vi "Self Configure.vi"(8 "error in":errorcluster, 11 "PowerSupply in":refnum<class "PowerSupply.lvclass">) -> (0 "error out":errorcluster, 3 "PowerSupply out":refnum<class "PowerSupply.lvclass">)   [LabVIEW 2019, in "PowerSupply.lvlib" / "PowerSupply.lvclass"]
uses:
  Library/PowerSupply.lvclass
  Custom Controls/Configuration Keys.ctl
  Library/PowerSupply.lvclass/PowerSupply.ctl
  builds/Instruments/Instruments.lvlibp/Library/Instruments.lvclass
  builds/Tools/Config.lvlibp/Config.lvclass
  C:/Users/Public/Documents/Development/builds/Instruments/Instruments.lvlibp/Library/Instruments.lvclass
  C:/Users/Public/Documents/Development/builds/Tools/Config.lvlibp/Config.lvclass
  C:/Users/Public/Documents/Development/builds/Engine/Engine.lvlibp/Project/Engine.lvclass
  C:/Users/Public/Documents/Development/builds/Engine/State Actor.lvlibp/Library/State Actor.lvclass
  C:/Users/Public/Documents/Development/builds/Engine/Panel Manager.lvlibp/Panel Actor/Panel Actor.lvclass
  C:/Users/Public/Documents/Development/builds/Engine/Monitored Actor.lvlibp/Monitored Actor/Monitored Actor/Monitored Actor.lvclass
  C:/Users/Public/Documents/Development/builds/Engine/Actor Framework.lvlibp/1abvi3w/vi.lib/ActorFramework/Actor/Actor.lvclass
panel:
  in  "Configuration Keys":T1
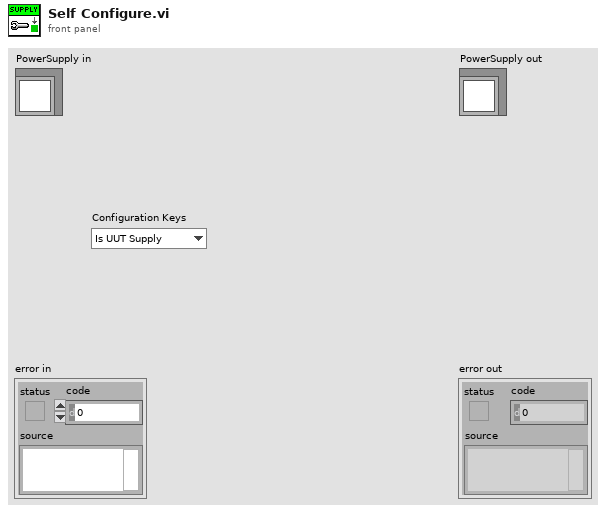
[diagram p1: front panel]
types:
  T1 = typedef "PowerSupply.lvlib/PowerSupply.lvclass/Configuration Keys.ctl" = enum16{"Is UUT Supply", "Number of Channels", "Channel Names", "Max Voltage", "Max Current", "Max OVP", "Max OCP", "Max Volt Ramp", "Max Curr Ramp"}
  T2 = typedef "PowerSupply.lvlib/PowerSupply.lvclass/Limits.ctl" = cluster{"Max_Current":dbl, "Max_Voltage":dbl, "Max_Current_Ramp":dbl, "Max_Voltage_Ramp":dbl, "Max_OCP":dbl, "Max_OVP":dbl}
  T3 = typedef "PowerSupply.lvlib/PowerSupply.lvclass/Settings.ctl" = cluster{"Voltage":dbl, "Current":dbl, "Output":bool, "OverVolt_Protect":dbl, "OverCurrent_Protect":dbl, "OVP":bool, "OCP":bool, "Interlock":bool, "Volt_Ramp":dbl, "Current_Ramp":dbl, "Sense Point":T4, "OCP Mode":T5, "Sharing":bool}
  T4 = typedef "PowerSupply.lvlib/PowerSupply.lvclass/Sense Point.ctl" = enum16{"Local", "Remote"}
  T5 = typedef "PowerSupply.lvlib/PowerSupply.lvclass/OCP Mode.ctl" = enum16{"Shutdown", "Foldback"}
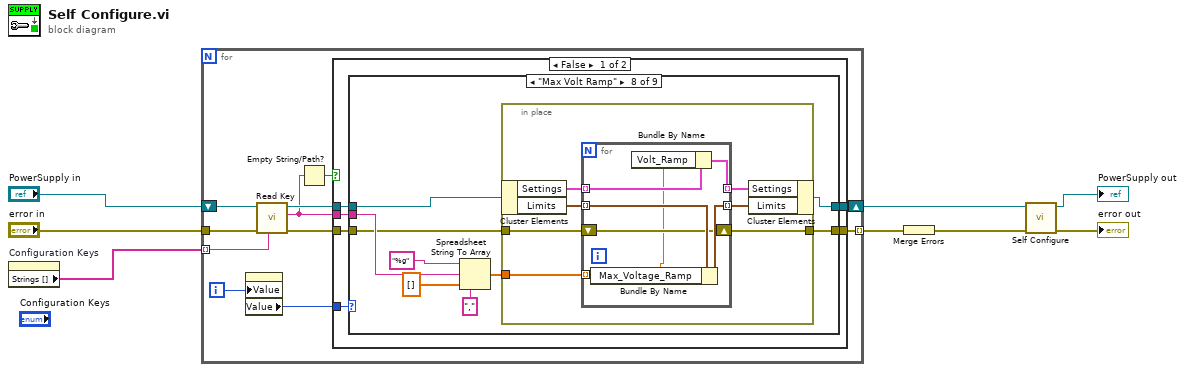
[diagram p0: block diagram]
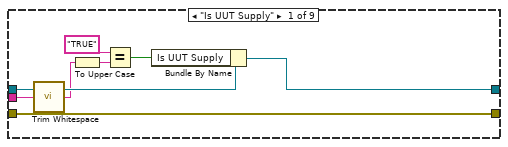
[diagram p2: hidden frame]
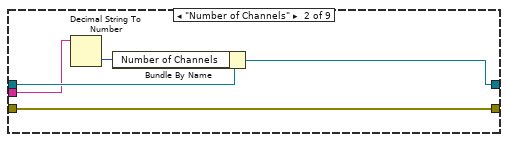
[diagram p3: hidden frame]
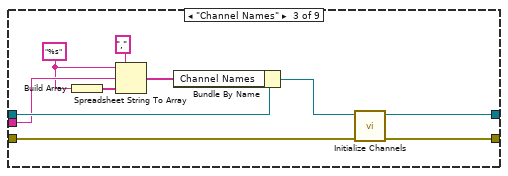
[diagram p4: hidden frame]
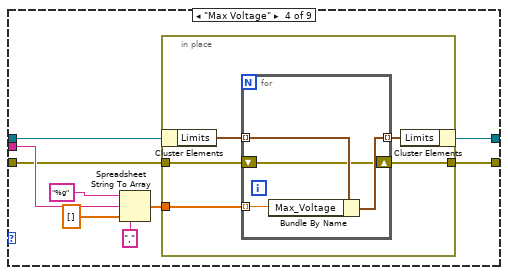
[diagram p5: hidden frame]
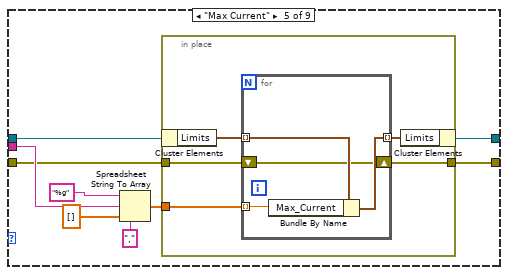
[diagram p6: hidden frame]
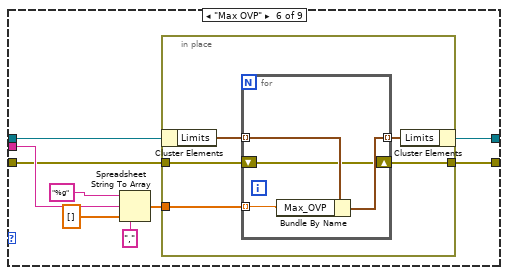
[diagram p7: hidden frame]
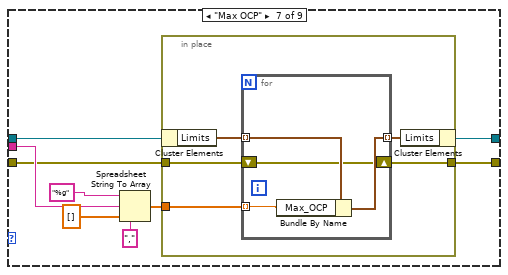
[diagram p8: hidden frame]
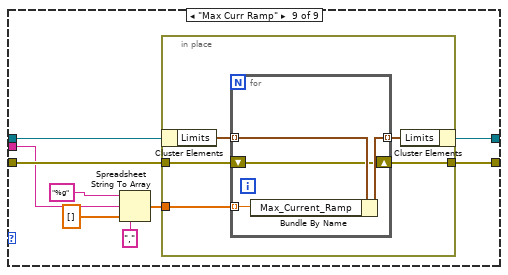
[diagram p9: hidden frame]
diagram:
  n1 = property on="Configuration Keys" class="Enum (strict)"() -> ("Strings []"=w8:string[])  [unwired: 2 in, 2 out]
  n2 = for {
    tunnel: w8 -> [w17] mode=indexing
    shift-right: [w13] -> w4
    shift-left: "PowerSupply in" -> [w19]
    tunnel: "error in" -> [w18]
    tunnel: [w14] -> w5 mode=indexing
    i -> [w12]
    n3 = property on="Configuration Keys" class="Enum (strict)"("Value"=w12) -> ("Value"=w11:T1)  [unwired: 2 in, 2 out]
    n4 = call "Read Key.vi"("Key Name"=w17, "error in"=w18, "Config in"=w19) -> ("error out"=w15:errorcluster, "Key Value"=w10:string, "Config out"=w16:refnum<class "PowerSupply.lvclass">)  [unwired: 6 in]
    n5 = Empty String/Path?(string/path=w10) -> (empty?=w9:bool)
    n6 = case shown="False" w9 {
      tunnel: w16 -> [w25 w162]
      tunnel: w15 -> [w24 w161]
      tunnel: [w23 w161] -> w14
      tunnel: [w22 w162] -> w13
      tunnel: w11 -> [w21 _]
      tunnel: w10 -> [w20 _]
      frame False {
        n7 = case shown="\"Max Volt Ramp\"" w21 {
          tunnel: w25 -> [w33 w38 w48 w53 w71 w89 w107 w125 w148]
          tunnel: w24 -> [w31 w34 w41 w50 w68 w86 w104 w122 w145]
          tunnel: w20 -> [w27 w37 w45 w56 w74 w92 w110 w128 w143]
          tunnel: [w31 w34 w40 w49 w67 w85 w103 w121 w144] -> w23
          tunnel: [w32 w35 w39 w52 w70 w88 w106 w124 w147] -> w22
          frame "Is UUT Supply" {
            n8 = call <vilib>:"Trim Whitespace.vi"("string"=w27) -> ("trimmed string"=w26:string)  [unwired: 1 in]
            n9 = To Upper Case(1:w26) -> (0:w28:string)
            n10 = Equal?(x="TRUE", y=w28) -> (x = y?=w29:bool)
            n11 = Bundle By Name(cluster=w33, "Is UUT Supply"=w29) -> (w32:refnum<class "PowerSupply.lvclass">)
          }
          frame "Number of Channels" {
            n12 = Decimal String To Number(string=w37) -> (number=w36:i32)  [unwired: 2 in, 1 out]
            n13 = Bundle By Name(cluster=w38, "Number of Channels"=w36) -> (w35:refnum<class "PowerSupply.lvclass">)
          }
          frame "Channel Names" {
            w44 = "%s" ("format string")
            n14 = Build Array(w44) -> (w47:string[])
            n15 = Spreadsheet String To Array(delimiter (Tab)=",", format string=w44, spreadsheet string=w45, array type (2D Dbl)=w47) -> (array=w43:string[])
            n16 = Bundle By Name(cluster=w48, "Channel Names"=w43) -> (w42:refnum<class "PowerSupply.lvclass">)
            n17 = call "Initialize Channels.vi"("error in"=w41, "PowerSupply in"=w42) -> ("error out"=w40:errorcluster, "PowerSupply out"=w39:refnum<class "PowerSupply.lvclass">)  [unwired: 8 in]
          }
          frame "Max Voltage" {
            n18 = Spreadsheet String To Array(delimiter (Tab)=",", format string="%g", spreadsheet string=w56, array type (2D Dbl)=dbl[] []) -> (array=w51:dbl[])
            n19 = in-place {
              in-place-border: w51 -> [w62]
              in-place-border: w50 -> [w59]
              in-place-border: [w58] -> w49
              n20 = in-place-cluster #1(w53) -> ("Limits"=w61:T2[])
              n21 = for {
                tunnel: w62 -> [w64] mode=indexing
                tunnel: w61 -> [w66] mode=indexing
                tunnel: [w65] -> w60 mode=indexing
                shift-right: [w63] -> w58
                shift-left: w59 -> [w63]
                n22 = Bundle By Name(cluster=w66, "Max_Voltage"=w64) -> (w65:T2)
              }
              n23 = in-place-cluster #1("Limits"=w60) -> (w52:refnum<class "PowerSupply.lvclass">)
            }
          }
          frame "Max Current" {
            n24 = Spreadsheet String To Array(delimiter (Tab)=",", format string="%g", spreadsheet string=w74, array type (2D Dbl)=dbl[] []) -> (array=w69:dbl[])
            n25 = in-place {
              in-place-border: w69 -> [w80]
              in-place-border: w68 -> [w77]
              in-place-border: [w76] -> w67
              n26 = in-place-cluster #2(w71) -> ("Limits"=w79:T2[])
              n27 = for {
                tunnel: w80 -> [w82] mode=indexing
                tunnel: w79 -> [w84] mode=indexing
                tunnel: [w83] -> w78 mode=indexing
                shift-right: [w81] -> w76
                shift-left: w77 -> [w81]
                n28 = Bundle By Name(cluster=w84, "Max_Current"=w82) -> (w83:T2)
              }
              n29 = in-place-cluster #2("Limits"=w78) -> (w70:refnum<class "PowerSupply.lvclass">)
            }
          }
          frame "Max OVP" {
            n30 = Spreadsheet String To Array(delimiter (Tab)=",", format string="%g", spreadsheet string=w92, array type (2D Dbl)=dbl[] []) -> (array=w87:dbl[])
            n31 = in-place {
              in-place-border: w87 -> [w98]
              in-place-border: w86 -> [w95]
              in-place-border: [w94] -> w85
              n32 = in-place-cluster #3(w89) -> ("Limits"=w97:T2[])
              n33 = for {
                tunnel: w98 -> [w100] mode=indexing
                tunnel: w97 -> [w102] mode=indexing
                tunnel: [w101] -> w96 mode=indexing
                shift-right: [w99] -> w94
                shift-left: w95 -> [w99]
                n34 = Bundle By Name(cluster=w102, "Max_OVP"=w100) -> (w101:T2)
              }
              n35 = in-place-cluster #3("Limits"=w96) -> (w88:refnum<class "PowerSupply.lvclass">)
            }
          }
          frame "Max OCP" {
            n36 = Spreadsheet String To Array(delimiter (Tab)=",", format string="%g", spreadsheet string=w110, array type (2D Dbl)=dbl[] []) -> (array=w105:dbl[])
            n37 = in-place {
              in-place-border: w105 -> [w116]
              in-place-border: w104 -> [w113]
              in-place-border: [w112] -> w103
              n38 = in-place-cluster #4(w107) -> ("Limits"=w115:T2[])
              n39 = for {
                tunnel: w116 -> [w118] mode=indexing
                tunnel: w115 -> [w120] mode=indexing
                tunnel: [w119] -> w114 mode=indexing
                shift-right: [w117] -> w112
                shift-left: w113 -> [w117]
                n40 = Bundle By Name(cluster=w120, "Max_OCP"=w118) -> (w119:T2)
              }
              n41 = in-place-cluster #4("Limits"=w114) -> (w106:refnum<class "PowerSupply.lvclass">)
            }
          }
          frame "Max Volt Ramp" {
            n42 = Spreadsheet String To Array(delimiter (Tab)=",", format string="%g", spreadsheet string=w128, array type (2D Dbl)=dbl[] []) -> (array=w123:dbl[])
            n43 = in-place {
              in-place-border: w123 -> [w136]
              in-place-border: w122 -> [w133]
              in-place-border: [w132] -> w121
              n44 = in-place-cluster #5(w125) -> ("Settings"=w131:T3[], "Limits"=w135:T2[])
              n45 = for {
                tunnel: w136 -> [w137] mode=indexing
                tunnel: w135 -> [w142] mode=indexing
                tunnel: [w141] -> w134 mode=indexing
                shift-right: [w140] -> w132
                shift-left: w133 -> [w140]
                tunnel: w131 -> [w139] mode=indexing
                tunnel: [w138] -> w130 mode=indexing
                n46 = Bundle By Name(cluster=w142, "Max_Voltage_Ramp"=w137) -> (w141:T2)
                n47 = Bundle By Name(cluster=w139, "Volt_Ramp"=w137) -> (w138:T3)
              }
              n48 = in-place-cluster #5("Settings"=w130, "Limits"=w134) -> (w124:refnum<class "PowerSupply.lvclass">)
            }
          }
          frame "Max Curr Ramp" {
            n49 = Spreadsheet String To Array(delimiter (Tab)=",", format string="%g", spreadsheet string=w143, array type (2D Dbl)=dbl[] []) -> (array=w146:dbl[])
            n50 = in-place {
              in-place-border: w146 -> [w156]
              in-place-border: w145 -> [w153]
              in-place-border: [w152] -> w144
              n51 = in-place-cluster #6(w148) -> ("Limits"=w155:T2[])
              n52 = for {
                tunnel: w156 -> [w158] mode=indexing
                tunnel: w155 -> [w160] mode=indexing
                tunnel: [w159] -> w154 mode=indexing
                shift-right: [w157] -> w152
                shift-left: w153 -> [w157]
                n53 = Bundle By Name(cluster=w160, "Max_Current_Ramp"=w158) -> (w159:T2)
              }
              n54 = in-place-cluster #6("Limits"=w154) -> (w147:refnum<class "PowerSupply.lvclass">)
            }
          }
        }
      }
      frame True {
      }
    }
  }
  n55 = Merge Errors(w5) -> (w3:errorcluster)
  n56 = call-parent "Self Configure.vi"("error in"=w3, "Instruments in"=w4) -> ("error out"=→"error out":errorcluster, "Instruments out"=→"PowerSupply out":refnum<class "PowerSupply.lvclass">)  [unwired: 8 in]
